vi "ReadHyperscopeINI_and_set_GFG.vi"(8 "error in (no error)":errorcluster) -> (0 "error out":errorcluster)   [LabVIEW 2012]
uses:
  <vilib>/Utility/config.llb/Read Key (Boolean).vi
  <vilib>/Utility/config.llb/Read Key (String).vi
  <vilib>/Utility/config.llb/NI_LVConfig.lvlib
panel:
  out "key names":string[][](array[string])
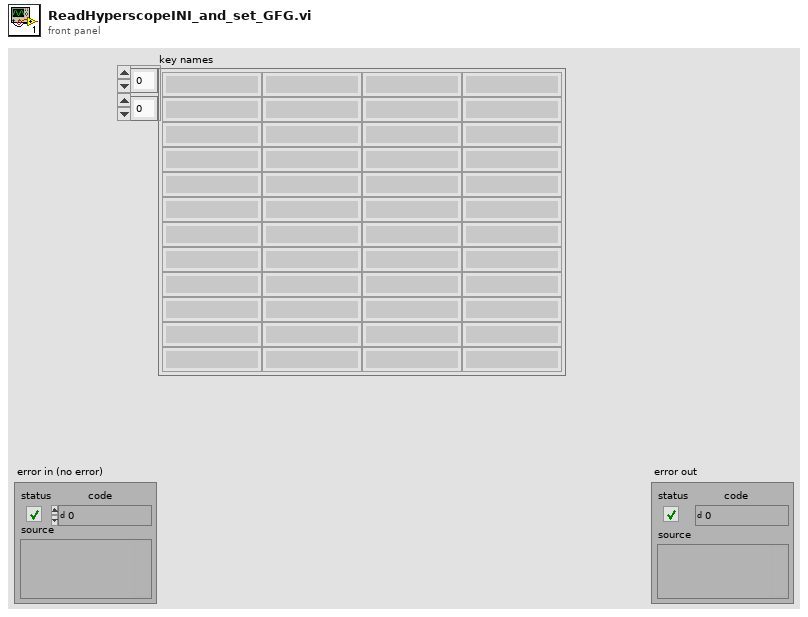
[diagram p1: front panel]
types:
  T1 = typedef "NI_LVConfig.lvlib/Config Data RefNum.ctl" = refnum<k1>
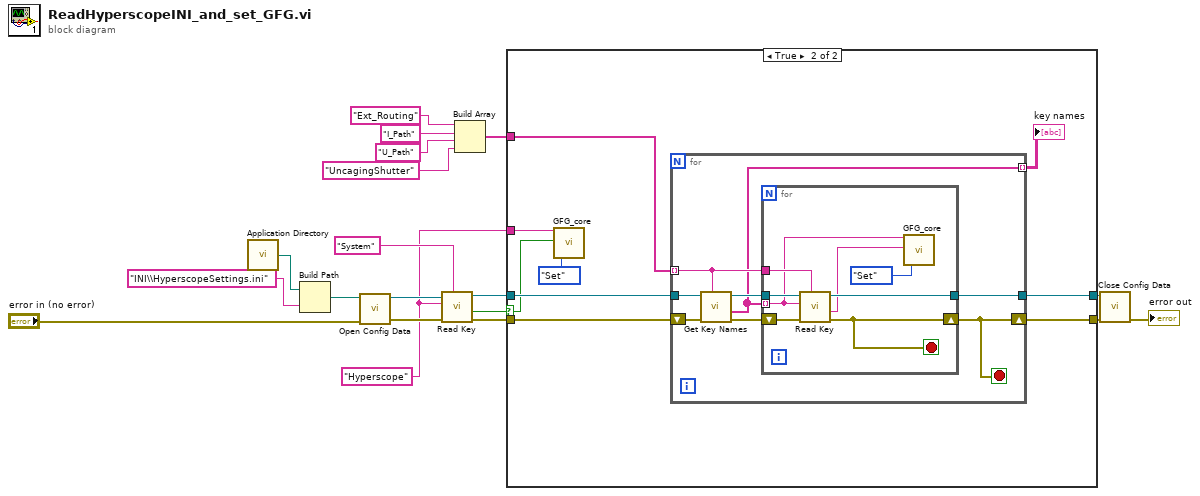
[diagram p0: block diagram]
diagram:
  w4 = "Hyperscope" ("key")
  n1 = call <vilib>:"Application Directory.vi"() -> ("Application Directory"=w14:path)
  n2 = Build Path(base path=w14, name or relative path="INI\\HyperscopeSettings.ini") -> (appended path=w16:path)
  n3 = call <vilib>:"Open Config Data.vi"("error in (no error)"="error in (no error)", "configuration file path"=w16) -> ("error out"=w19:errorcluster, "refnum"=w17:T1)  [unwired: 7 in, 1 out]
  n4 = call-poly <vilib>:"Read Key.vi"("section"="System", "error in (no error)"=w19, "key"=w4, "refnum"=w17) -> ("error out"=w10:errorcluster, "value"=w5:bool, "refnum out"=w9:T1)  [unwired: 4 in, 1 out]
  n5 = Build Array("Ext_Routing" ("section"), "I_Path" ("section"), "U_Path" ("section"), "UncagingShutter" ("section")) -> (w11:string[])
  n6 = case shown="True" w5 {
    selector: w5 -> [_ w23]
    tunnel: w11 -> [_ w30]
    tunnel: w10 -> [w21 w29]
    tunnel: w9 -> [w20 w28]
    tunnel: [w20 w27] -> w8
    tunnel: [w21 w26] -> w7
    tunnel: w4 -> [_ w24]
    frame False {
    }
    frame True {
      n7 = call "GFG_core.vi"("Variable Name in"=w24, "Variant in"=w23, "Action"=enum16{"Init", "Set", "Get", "Clear"}."Set") -> ()  [unwired: 10 in, 7 out]
      n8 = for {
        tunnel: w30 -> [w38] mode=indexing
        shift-right: [w32] -> w26
        shift-left: w29 -> [w36]
        tunnel: w28 -> [w35]
        tunnel: [w33] -> w27
        tunnel: [w31] -> w22 mode=indexing
        stop <- w32 stop-if-true
        n9 = call <vilib>:"Get Key Names.vi"("section"=w38, "error in (no error)"=w36, "refnum"=w35) -> ("error out"=w37:errorcluster, "key names"=w31:string[], "refnum out"=w34:T1)  [unwired: 5 in, 1 out]
        n10 = for {
          tunnel: w38 -> [w46]
          tunnel: w31 -> [w40] mode=indexing
          shift-right: [w42] -> w32
          shift-left: w37 -> [w45]
          tunnel: w34 -> [w44]
          tunnel: [w43] -> w33
          stop <- w42 stop-if-true
          n11 = call-poly <vilib>:"Read Key.vi"("section"=w46, "error in (no error)"=w45, "key"=w40, "refnum"=w44) -> ("error out"=w42:errorcluster, "value"=w39:string, "refnum out"=w43:T1)  [unwired: 4 in, 1 out]
          n12 = call "GFG_core.vi"("Variable Name in"=w40, "Variant in"=w39, "Action"=enum16{"Init", "Set", "Get", "Clear"}."Set") -> ()  [unwired: 10 in, 7 out]
        }
      }
      "key names" <- w22
    }
  }
  n13 = call <vilib>:"Close Config Data.vi"("error in (no error)"=w7, "refnum"=w8) -> ("error out"=→"error out":errorcluster)  [unwired: 8 in, 1 out]
